vi ".NET Type Builder Define Module.vi"(8 "error in (no error)":errorcluster, 9 ".NET Assembly Builder":refnum<k24>, 10 "Name":string) -> (0 "error out":errorcluster, 1 ".NET Module Builder":refnum<k24>)   [LabVIEW 2018, in "TwinCAT ADS.lvclass"]
uses:
  TwinCAT ADS.lvclass
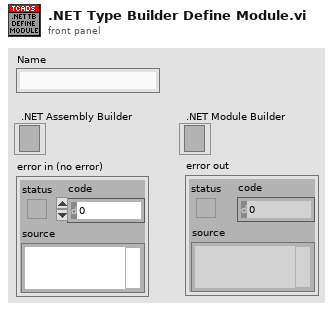
[diagram p1: front panel]
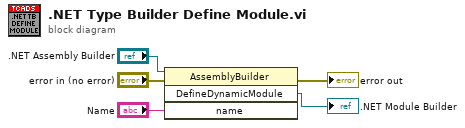
[diagram p0: block diagram]
diagram:
  n1 = invoke class="AssemblyBuilder" method="DefineDynamicModule"(reference=".NET Assembly Builder", error in="error in (no error)", "name"="Name") -> (error out=→"error out":errorcluster, "DefineDynamicModule"=→".NET Module Builder":refnum<k24>)  [unwired: 1 in, 2 out]
